vi "InitCameraPoly.vi"   [LabVIEW 2024]
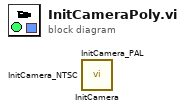
[diagram p0: block diagram]
diagram:
  n1 = call <userlib>:"InitCamera.vi"() -> ()  [unwired: 2 in, 2 out]
  n2 = call <userlib>:"InitCamera_PAL.vi"() -> ()  [unwired: 2 in, 2 out]
  n3 = call <userlib>:"InitCamera_NTSC.vi"() -> ()  [unwired: 2 in, 2 out]
